vi "SnakeGrowth.vi"(9 "Key input":T1, 10 "Level input":u32[][](array[colorbox]), 11 "Location input":cluster{"Y":i32, "X":i32}[](array[cluster])=[{"Y"=12, "X"=8}, {"Y"=12, "X"=7}, {"Y"=12, "X"=6}, {"Y"=12, "X"=5}]) -> (1 "Key output":T1, 2 "Level output":u32[][](array[colorbox]), 3 "Location output":cluster{"Y":i32, "X":i32}[](array[cluster])=[{"Y"=12, "X"=8}, {"Y"=12, "X"=7}, {"Y"=12, "X"=6}, {"Y"=12, "X"=5}])   [LabVIEW 2021]
uses:
  TypeDef/KeyDown.ctl
  GlobalVariables/Board_Colors.vi
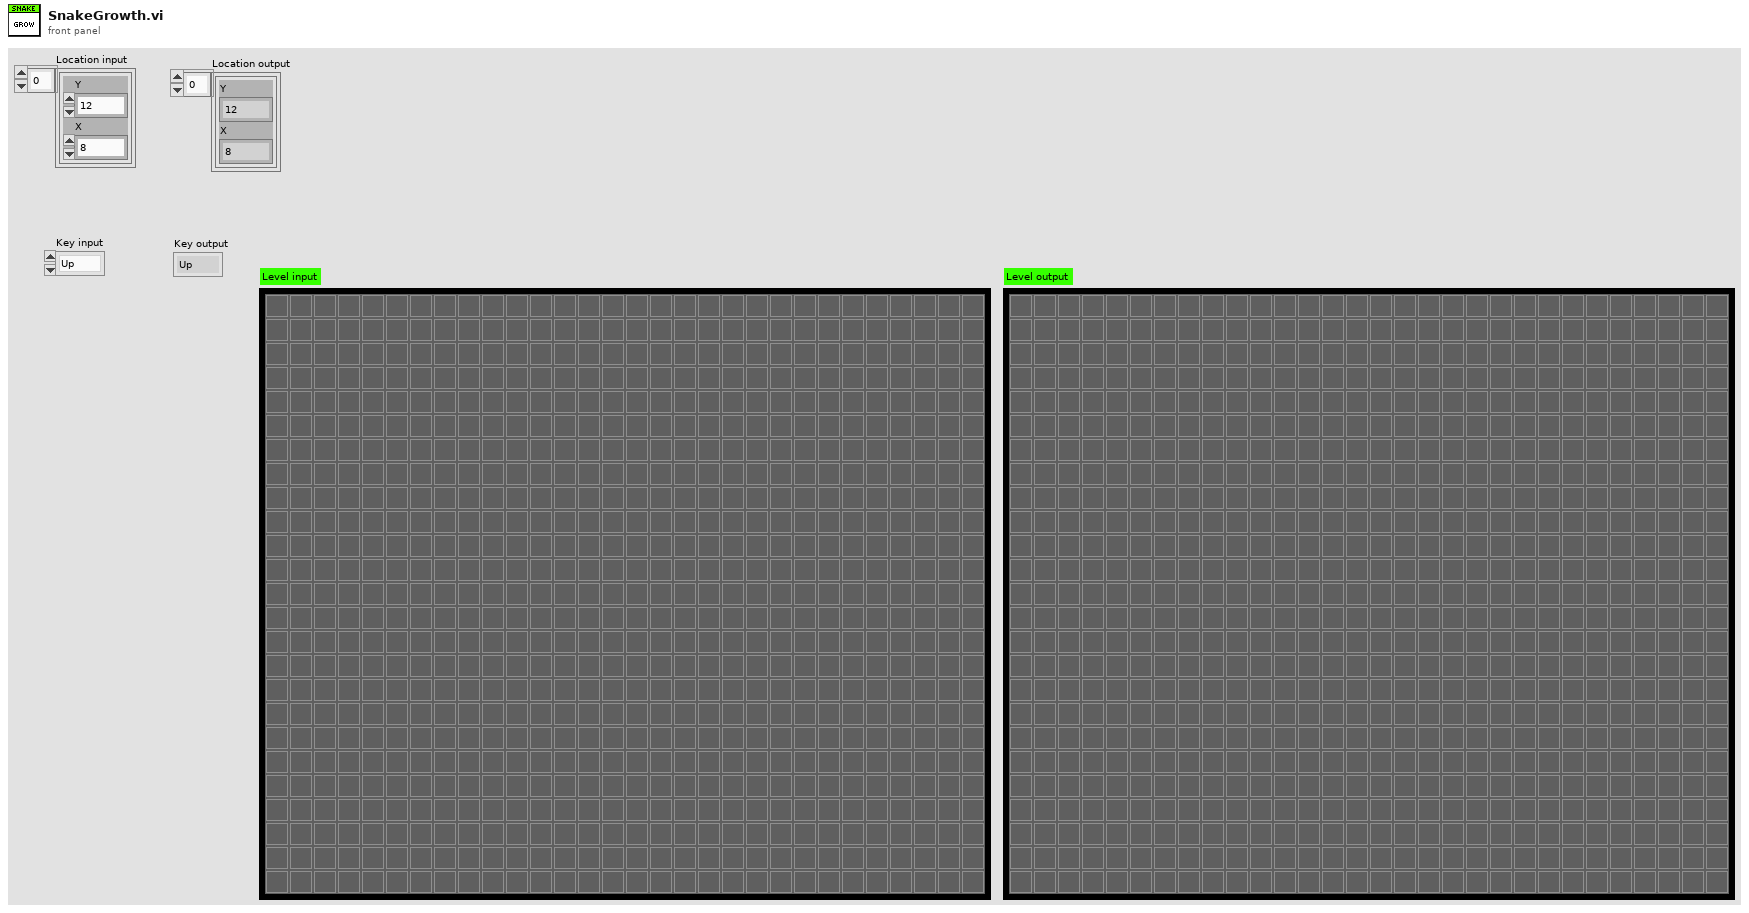
[diagram p1: front panel]
types:
  T1 = typedef "KeyDown.ctl" = enum16{"Up", "Down", "Left", "Right"}
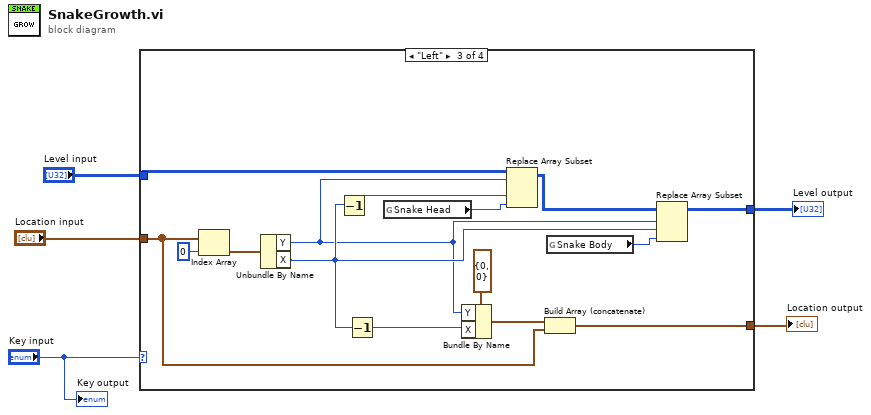
[diagram p0: block diagram]
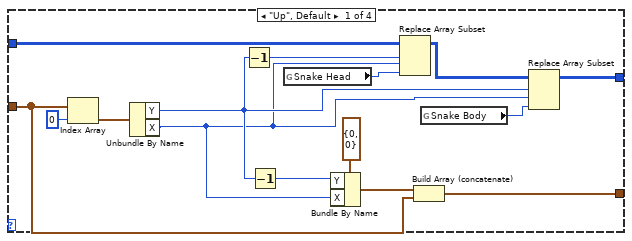
[diagram p2: hidden frame]
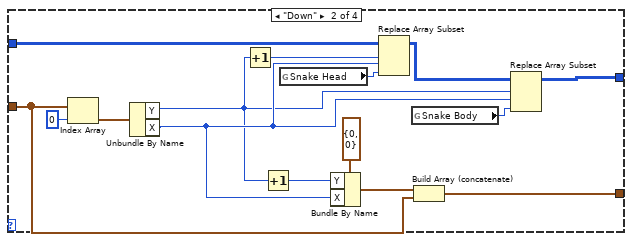
[diagram p3: hidden frame]
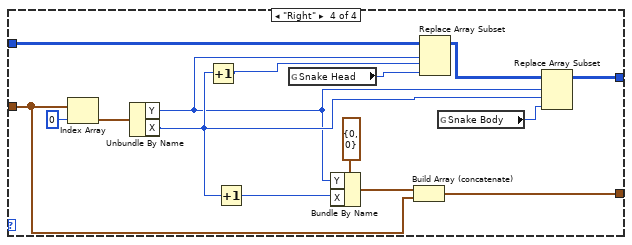
[diagram p4: hidden frame]
diagram:
  n1 = case shown="\"Left\"" "Key input" {
    tunnel: "Location input" -> [w12 w31 w45 w60]
    tunnel: "Level input" -> [w18 w26 w48 w63]
    tunnel: [w16 w32 w46 w61] -> w2
    tunnel: [w9 w28 w42 w57] -> w1
    frame "Up", Default {
      n2 = Index Array(array=w12, index=0) -> (element=w19:cluster{"Y":i32, "X":i32})
      n3 = Unbundle By Name(w19) -> ("Y"=w13:i32, "X"=w8:i32)
      n4 = Decrement(x=w13) -> (x-1=w15:i32)
      n5 = Decrement(x=w13) -> (x-1=w14:i32)
      n6 = global read "Board_Colors.vi" "Snake Head"() -> (w7:u32)
      n7 = Bundle By Name(cluster=cluster{"Y":i32, "X":i32} {"Y"=0, "X"=0} ("input cluster"), "Y"=w14, "X"=w8) -> (w10:cluster{"Y":i32, "X":i32})
      n8 = Replace Array Subset(array=w18, new element=w7, index (row)=w15, index (col)=w8) -> (w17:u32[][])
      n9 = Build Array (concatenate)(w10, w12) -> (w9:cluster{"Y":i32, "X":i32}[])
      n10 = global read "Board_Colors.vi" "Snake Body"() -> (w6:u32)
      n11 = Replace Array Subset(array=w17, new element=w6, index (row)=w13, index (col)=w8) -> (w16:u32[][])
    }
    frame "Down" {
      n12 = Index Array(array=w31, index=0) -> (element=w34:cluster{"Y":i32, "X":i32})
      n13 = Unbundle By Name(w34) -> ("Y"=w21:i32, "X"=w27:i32)
      n14 = Increment(x=w21) -> (x+1=w22:i32)
      n15 = Increment(x=w21) -> (x+1=w23:i32)
      n16 = global read "Board_Colors.vi" "Snake Head"() -> (w24:u32)
      n17 = Bundle By Name(cluster=cluster{"Y":i32, "X":i32} {"Y"=0, "X"=0} ("input cluster"), "Y"=w23, "X"=w27) -> (w29:cluster{"Y":i32, "X":i32})
      n18 = Replace Array Subset(array=w26, new element=w24, index (row)=w22, index (col)=w27) -> (w33:u32[][])
      n19 = global read "Board_Colors.vi" "Snake Body"() -> (w25:u32)
      n20 = Build Array (concatenate)(w29, w31) -> (w28:cluster{"Y":i32, "X":i32}[])
      n21 = Replace Array Subset(array=w33, new element=w25, index (row)=w21, index (col)=w27) -> (w32:u32[][])
    }
    frame "Left" {
      n22 = Index Array(array=w45, index=0) -> (element=w49:cluster{"Y":i32, "X":i32})
      n23 = Unbundle By Name(w49) -> ("Y"=w38:i32, "X"=w39:i32)
      n24 = Decrement(x=w39) -> (x-1=w41:i32)
      n25 = Decrement(x=w39) -> (x-1=w40:i32)
      n26 = global read "Board_Colors.vi" "Snake Head"() -> (w36:u32)
      n27 = Bundle By Name(cluster=cluster{"Y":i32, "X":i32} {"Y"=0, "X"=0} ("input cluster"), "Y"=w38, "X"=w40) -> (w43:cluster{"Y":i32, "X":i32})
      n28 = Replace Array Subset(array=w48, new element=w36, index (row)=w38, index (col)=w41) -> (w47:u32[][])
      n29 = Build Array (concatenate)(w43, w45) -> (w42:cluster{"Y":i32, "X":i32}[])
      n30 = global read "Board_Colors.vi" "Snake Body"() -> (w37:u32)
      n31 = Replace Array Subset(array=w47, new element=w37, index (row)=w38, index (col)=w39) -> (w46:u32[][])
    }
    frame "Right" {
      n32 = Index Array(array=w60, index=0) -> (element=w64:cluster{"Y":i32, "X":i32})
      n33 = Unbundle By Name(w64) -> ("Y"=w53:i32, "X"=w54:i32)
      n34 = Increment(x=w54) -> (x+1=w56:i32)
      n35 = Increment(x=w54) -> (x+1=w55:i32)
      n36 = global read "Board_Colors.vi" "Snake Head"() -> (w51:u32)
      n37 = Bundle By Name(cluster=cluster{"Y":i32, "X":i32} {"Y"=0, "X"=0} ("input cluster"), "Y"=w53, "X"=w55) -> (w58:cluster{"Y":i32, "X":i32})
      n38 = Build Array (concatenate)(w58, w60) -> (w57:cluster{"Y":i32, "X":i32}[])
      n39 = Replace Array Subset(array=w63, new element=w51, index (row)=w53, index (col)=w56) -> (w62:u32[][])
      n40 = global read "Board_Colors.vi" "Snake Body"() -> (w52:u32)
      n41 = Replace Array Subset(array=w62, new element=w52, index (row)=w53, index (col)=w54) -> (w61:u32[][])
    }
  }
  "Level output" <- w2
  "Location output" <- w1
  "Key output" <- "Key input"
